vi "Create Groups in Memory.vi"(8 "error in (no error)":errorcluster, 11 "Group Listings":T1[](array[typedef])) -> (0 "error out":errorcluster)   [LabVIEW 2010, in "Current Value Table.lvlib"]
doc: "This VI takes a set of groups and generates all of them in memory."
uses:
  Current Value Table.lvlib
  Type Defs/Tag Grouping set.ctl
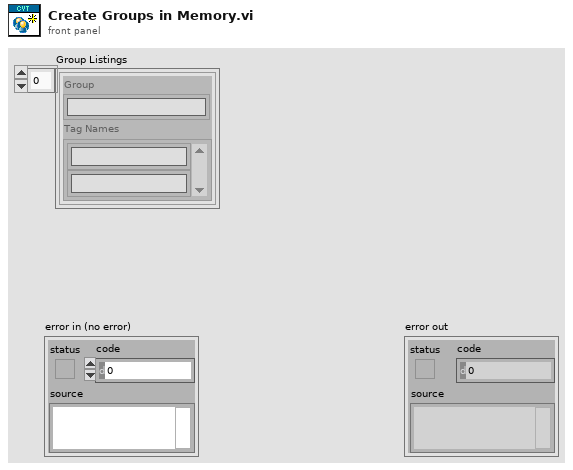
[diagram p1: front panel]
types:
  T1 = typedef "Current Value Table.lvlib/Tag Grouping set.ctl" = cluster{"Group":string, "Tag Names":string[]}
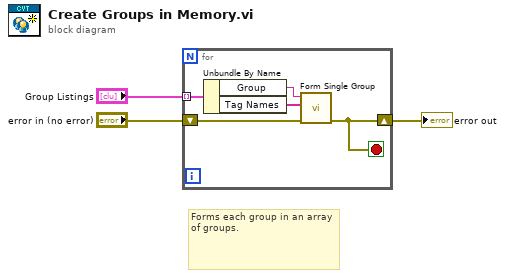
[diagram p0: block diagram]
diagram:
  # "Forms each group in an array of groups."
  n1 = for {
    tunnel: "Group Listings" -> [w8] mode=indexing
    shift-right: [w5] -> w3
    shift-left: "error in (no error)" -> [w4]
    stop <- w5 stop-if-true
    n2 = Unbundle By Name(w8) -> ("Group"=w7:string, "Tag Names"=w6:string[])
    n3 = call "Form Single Group.vi"("error in (no error)"=w4, "Names"=w6, "Group"=w7) -> ("error out"=w5:errorcluster)  [unwired: 8 in]
  }
  "error out" <- w3
